vi "Finish Measurement.vi"(8 "error in (no error)":errorcluster, 11 "XML Handler in":refnum<class "XML Handler.lvclass">) -> (0 "error out":errorcluster, 3 "XML Handler out":refnum<class "XML Handler.lvclass">)   [LabVIEW 2020, in "XML Handler.lvclass"]
uses:
  XML Handler.lvclass
  XML Handler.lvclass/XML Handler.ctl
  <vilib>/xml/Close Reference(Node).vi
  <resource>/objmgr/DOMUserDefRef.rc
  <vilib>/xml/NI_XML.lvlib
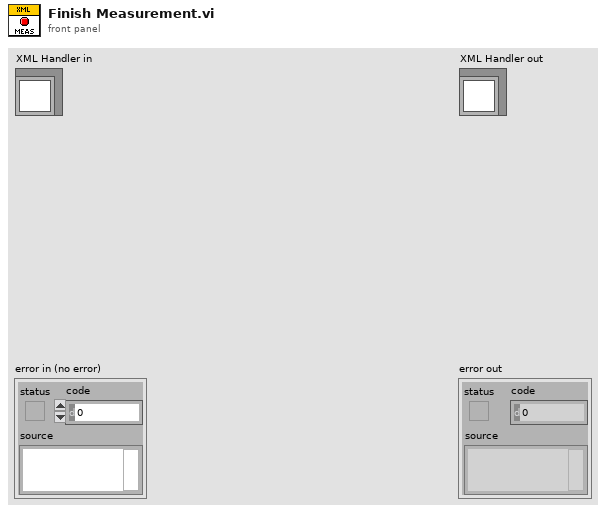
[diagram p1: front panel]
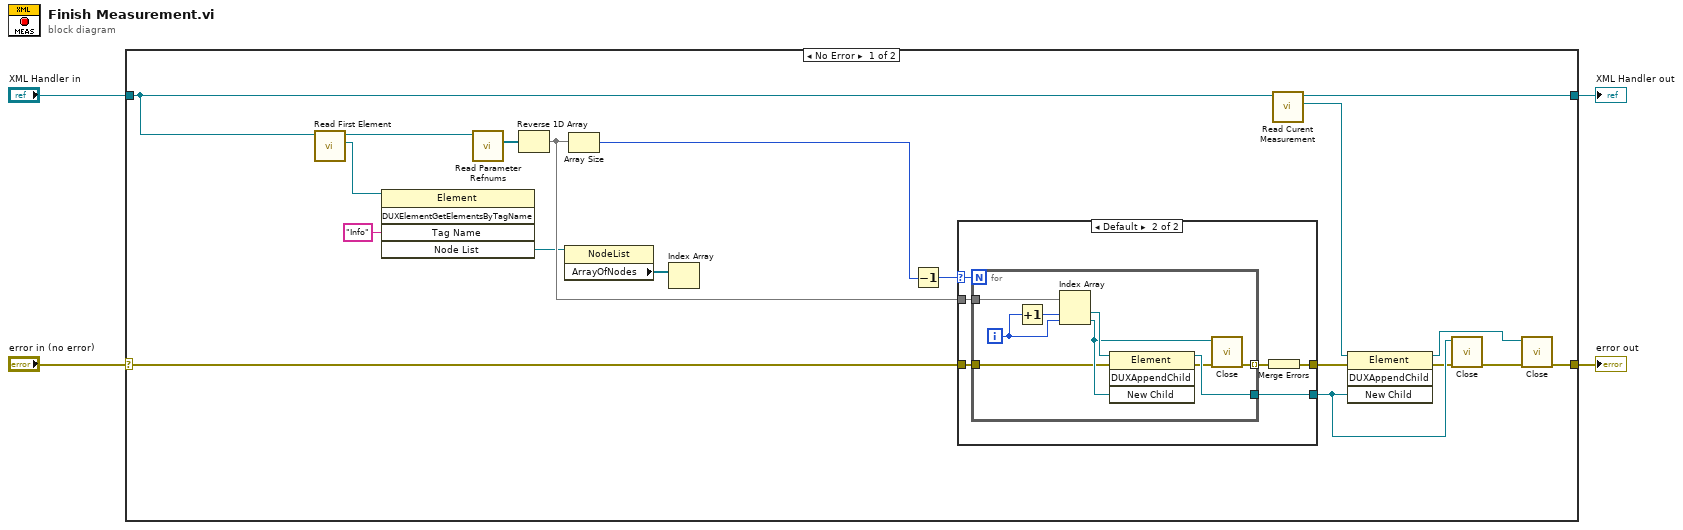
[diagram p0: block diagram]
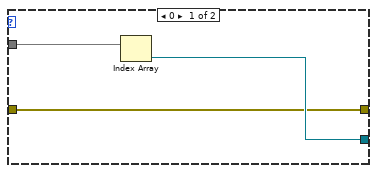
[diagram p2: hidden frame]
diagram:
  n1 = case shown="No Error" "error in (no error)" {
    selector: "error in (no error)" -> [w5 w43]
    tunnel: [w13 w43] -> w3
    tunnel: [w16 w42] -> w1
    tunnel: "XML Handler in" -> [w10 w42]
    frame No Error {
      n2 = call "Read First Element.vi"("XML Handler in"=w10) -> ("First Element"=w8:refnum<k20>, "XML Handler out"=w11:refnum<class "XML Handler.lvclass">)  [unwired: 9 in]
      n3 = invoke class="Element" method="DUXElementGetElementsByTagName"(reference=w8, "Tag Name"="Info") -> ("Node List"=w6:refnum<k20>)  [unwired: 3 in, 4 out]
      n4 = call "Read Parameter Refnums.vi"("XML Handler in"=w11) -> ("Parameter Refnums"=w23:refnum<k20>[])  [unwired: 9 in, 1 out]
      n5 = Reverse 1D Array(array=w23) -> (reversed array=w21:refnum<k20>[])
      n6 = property class="NodeList"(reference=w6) -> ("ArrayOfNodes"=w7:refnum<k20>[])  [unwired: 1 in, 2 out]
      n7 = Array Size(array=w21) -> (size(s)=w22:i32)
      n8 = Index Array(array=w7) -> ()  [unwired: 1 in, 1 out]
      n9 = Decrement(x=w22) -> (x-1=w14:i32)
      n10 = case shown="Default" w14 {
        selector: w14 -> [_ w27]
        tunnel: w21 -> [w26 w32]
        tunnel: [w25 w31] -> w19
        tunnel: [w24 w28] -> w12
        tunnel: w5 -> [w24 w30]
        frame 0 {
          n11 = Index Array(array=w26) -> (element=w25:refnum<k20>)  [unwired: 1 in]
        }
        frame Default {
          n12 = for {
            N: w27 -> [_]
            tunnel: w32 -> [w41]
            tunnel: [w37] -> w31
            tunnel: [w34] -> w29 mode=indexing
            tunnel: w30 -> [w33]
            i -> [w39]
            n13 = Increment(x=w39) -> (x+1=w40:i32)
            n14 = Index Array(array=w41, index #1=w40, index #2=w39) -> (element #1=w38:refnum<k20>, element #2=w35:refnum<k20>)
            n15 = invoke class="Element" method="DUXAppendChild"(reference=w38, error in=w33, "New Child"=w35) -> (reference out=w37:refnum<k20>, error out=w36:errorcluster)  [unwired: 1 in, 2 out]
            n16 = call-poly <vilib>:"Close.vi"("error in (no error)"=w36, "node"=w35) -> ("error out"=w34:errorcluster)  [unwired: 7 in]
          }
          n17 = Merge Errors(w29) -> (w28:errorcluster)
        }
      }
      n18 = call "Read Curent Measurement.vi"("XML Handler in"=w10) -> ("Curent Measurement"=w20:refnum<k20>, "XML Handler out"=w16:refnum<class "XML Handler.lvclass">)  [unwired: 9 in]
      n19 = invoke class="Element" method="DUXAppendChild"(reference=w20, error in=w12, "New Child"=w19) -> (reference out=w17:refnum<k20>, error out=w18:errorcluster)  [unwired: 1 in, 2 out]
      n20 = call-poly <vilib>:"Close.vi"("error in (no error)"=w18, "node"=w19) -> ("error out"=w15:errorcluster)  [unwired: 7 in]
      n21 = call-poly <vilib>:"Close.vi"("error in (no error)"=w15, "node"=w17) -> ("error out"=w13:errorcluster)  [unwired: 7 in]
    }
    frame Error {
    }
  }
  "error out" <- w3
  "XML Handler out" <- w1
